vi "LaguerrePolynomial.vi"(1 "a":i16, 2 "n":i16, 3 "x":dbl format="%.2f") -> (0 "associated Laguerre polynomial (n,a,x)":dbl format="%.2f")   [LabVIEW 2024]
uses:
  <vilib>/gmath/NI_Gmath.lvlib
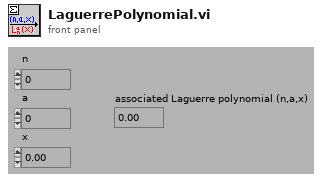
[diagram p1: front panel]
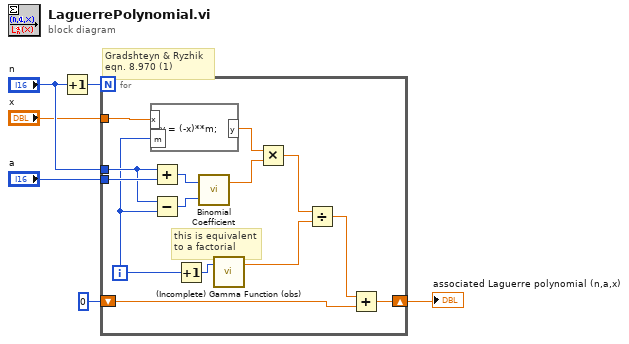
[diagram p0: block diagram]
diagram:
  # "Gradshteyn & Ryzhik\neqn. 8.970 (1)"
  n1 = Increment(x="n") -> (x+1=w6:i16)
  n2 = for {
    N: w6 -> [_]
    shift-right: [w12] -> w1
    shift-left: 0 -> [w8]
    tunnel: "x" -> [w20]
    tunnel: "a" -> [w19]
    tunnel: "n" -> [w17]
    i -> [w11]
    # "this is equivalent\nto a factorial"
    n3 = formula code="y = (-x)**m;"("x"=w20, "m"=w11) -> ("y"=w15:dbl)
    n4 = Add(x=w17, y=w19) -> (x+y=w18:i16)
    n5 = Subtract(x=w17, y=w11) -> (x-y=w16:i32)
    n6 = Increment(x=w11) -> (x+1=w7:i32)
    n7 = call <vilib>:"Binomial Coefficient.vi"("k"=w16, "n"=w18) -> ("binomial coefficient (n,k)"=w14:dbl)  [unwired: 1 out]
    n8 = call <vilib>:"(Incomplete) Gamma Function (obs).vi"("x"=w7) -> ("g(x, a)"=w10:dbl)  [unwired: 2 in]
    n9 = Multiply(x=w15, y=w14) -> (x*y=w13:dbl)
    n10 = Divide(x=w13, y=w10) -> (x/y=w9:dbl)
    n11 = Add(x=w9, y=w8) -> (x+y=w12:dbl)
  }
  "associated Laguerre polynomial (n,a,x)" <- w1
